vi "ClusterModificationMarcoGonzalez.vi"() -> ()   [LabVIEW 2012]
doc: "1) The VI allows the user to input the following items into Cluster 1: A numeric, 2 boolean switches and a slide input\n2) Inputs that allow you to modify 2 of the 4 items \n3) A modified Cluster ouput that displays all 4 items (2 should be modified)\n4) A small cluster that includes the 2 items you did not modify"
panel:
  in  "stop":bool
  out "Output (Non-Modified)":cluster{"Norwegian?":bool, "PC Gemer?":bool}
  out "Output":T1
  in  "Do you like chocolate pie?":bool
  in  "# of Years Living in the Intercontinental U.S":dbl
  in  "Input":T2
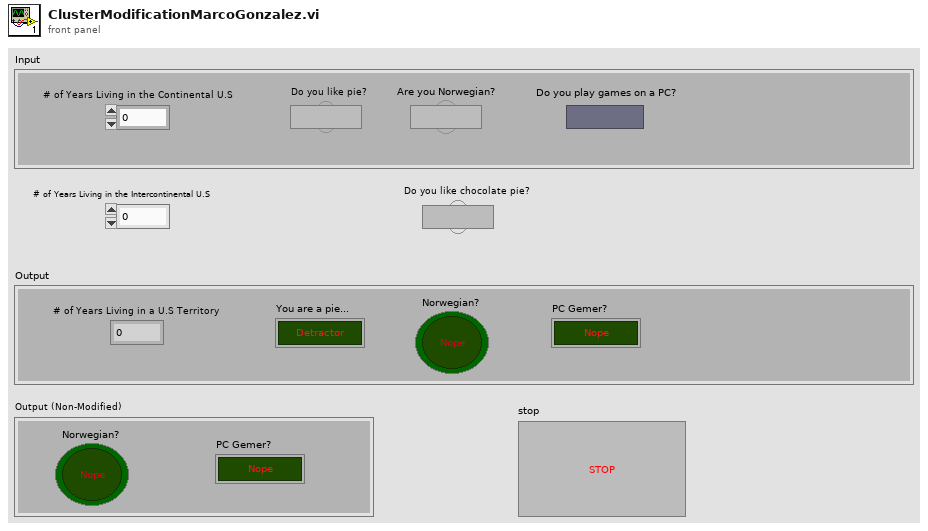
[diagram p1: front panel]
types:
  T1 = cluster{"# of Years Living in a U.S Territory":dbl, "You are a pie...":bool, "Norwegian?":bool, "PC Gemer?":bool}
  T2 = cluster{"# of Years Living in the Continental U.S":dbl, "Do you like pie?":bool, "Are you Norwegian?":bool, "Do you play games on a PC?":bool}
  T3 = cluster{"Are you Norwegian?":bool, "Do you play games on a PC?":bool}
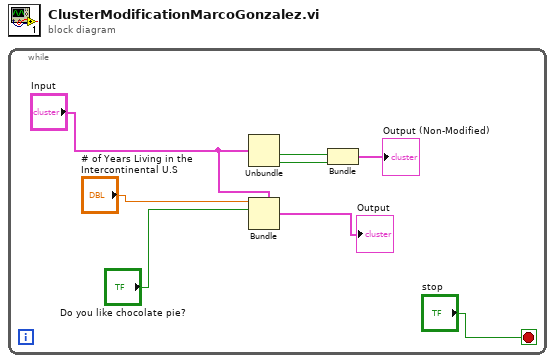
[diagram p0: block diagram]
diagram:
  n1 = while {
    stop <- "stop" stop-if-true
    n2 = Unbundle("Input") -> ("Are you Norwegian?"=w5:bool, "Do you play games on a PC?"=w4:bool)  [unwired: 2 out]
    n3 = Bundle(cluster="Input", "# of Years Living in the Continental U.S"="# of Years Living in the Intercontinental U.S", "Do you like pie?"="Do you like chocolate pie?") -> (→"Output":T2)  [unwired: 2 in]
    n4 = Bundle("Are you Norwegian?"=w5, "Do you play games on a PC?"=w4) -> (→"Output (Non-Modified)":T3)  [unwired: 1 in]
  }
